vi "Get Module Info.vi"(0 "IO Container":refnum<k21> caption="IO容器", 3 "error in (no error)":errorcluster caption="错误输入（无错误）") -> (7 "IO Container(dup)":refnum<k21> caption="IO容器（副本）", 8 "channel info array":cluster{"Module":string, "Channel":string}[](array[cluster]) caption="通道信息数组", 10 "error out":errorcluster caption="错误输出")   [LabVIEW 2015]
uses:
  <resource>/objmgr/ni.var.rc
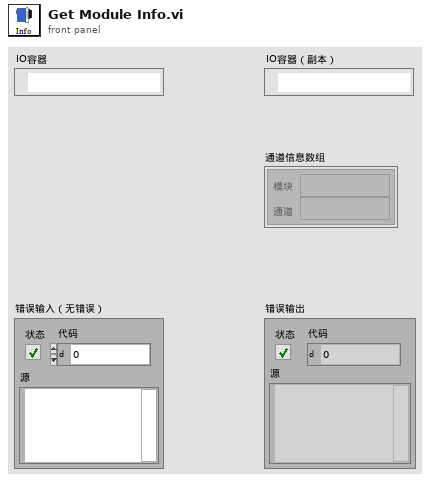
[diagram p1: front panel]
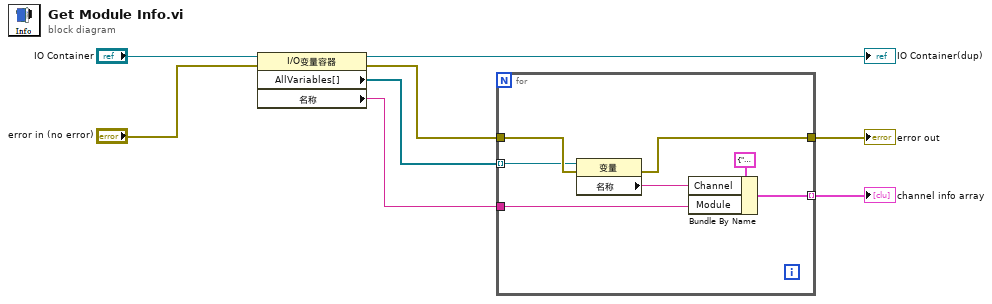
[diagram p0: block diagram]
diagram:
  n1 = property class="I/O变量容器"(reference="IO Container", error in="error in (no error)") -> (reference out=→"IO Container(dup)":refnum<k21>, error out=w7:errorcluster, "AllVariables[]"=w3:refnum<k21>[], "名称"=w2:string)
  n2 = for {
    tunnel: [w15] -> w8
    tunnel: w7 -> [w14]
    tunnel: w3 -> [w13] mode=indexing
    tunnel: w2 -> [w11]
    tunnel: [w10] -> w1 mode=indexing
    n3 = property class="变量"(reference=w13, error in=w14) -> (error out=w15:errorcluster, "名称"=w12:string)  [unwired: 1 out]
    n4 = Bundle By Name(cluster=cluster{"Module":string, "Channel":string} {"Module"="", "Channel"=""} ("Acquisition Info"), "Channel"=w12, "Module"=w11) -> (w10:cluster{"Module":string, "Channel":string})
  }
  "error out" <- w8
  "channel info array" <- w1
